vi "Laser.vi"() -> ()   [LabVIEW 2013]
doc: "Пограмма управления мишенью лазерного источника ионов."
uses:
  <vilib>/Utility/error.llb/DialogType.ctl
  <vilib>/Utility/inputDevices.llb/closeMouse.vi
  <vilib>/Utility/inputDevices.llb/mouseAcquire.vi
panel:
  in  "выстрел  Y Графит":u16 step=1
  in  "выстрел X Графит":u16 step=1
  in  "выстрел Y LiF 2":u16 step=1
  in  "выстрел X LiF 2":u16 step=1
  in  "выстрел Y LiF 1":u16 step=1
  in  "выстрел X LiF 1":u16 step=1
  in  "выстрел Y дейт":u16 step=1
  in  "выстрел X дейт":u16 step=1
  in  "xxx":enum32{" Мишени", " Настройки TCP"}(tab)
  in  "Готово!":bool
  in  "Выстрелов до перемотки":u16=5
  out "id мишени":u16
  in  "Выбор - дейтерий":bool
  in  "Счетчик выстрелов:":dbl
  in  "Шаг перехода по Y графит":dbl format="%.1g"
  in  "Шаг перехода по Х графит":dbl format="%.1g"
  in  "Выстрелов в точку  графит":u16=3
  in  "Шаг перехода по Y LiF 2":dbl format="%.1g"
  in  "Шаг перехода по Х LiF 2":dbl format="%.1g"
  in  "Выстрелов в точку  LiF 2":u16=3
  in  "Шаг перехода по Y LiF 1":dbl format="%.1g"
  in  "Шаг перехода по Х LiF 1":dbl format="%.1g"
  in  "Выстрелов в точку LiF 1":u16=3
  in  "Шаг перехода по Y дейт":dbl format="%.1g"
  in  "Шаг перехода по Х дейт":dbl format="%.1g"
  in  "Выстрелов в точку дейтерий":u16=3
  in  "TCP read data":string
  in  "LiF 2":picture
  in  "LiF 1":picture
  in  "Графит":picture
  in  "Дейтерий":picture
  out "Slide X axis":u8(slide) max=100 scale=0.0..100.0
  out "Slide Y axis":u8(slide) max=50 step=1
  in  "Снимок":bool
  out "con err":bool caption="Connect"
  out "Con":bool
  out "warning1":string
  out "Mouse on Pane pos Horizontal":i32
  out "Mouse on Pane pos Vertical":i32
  in  "Выбор - LiF 1":bool
  in  "Выбор - LiF 2":bool
  in  "Выбор -  Графит":bool
  in  "Выстрел по мишени!":u32
  in  "порт":u16=10001
  in  "IP-адрес":string="159.93.126.157"
  in  "Disconnect":bool caption="Disconn"
  out "Connected":bool
  in  "Connect":bool
  out "TCP error source":string
  in  "stop":bool
  out "read_error_indicator":bool
  in  "Connect 2":bool caption="Connect"
  in  "flag1":bool caption="Disconn"
  out "x+1":dbl
  out "TCP con ID":refnum<k5>
  # "LiF 1"
  # "Дейтерированный полиэтилен"
  # "LiF 2"
  # "Графит"
  # "Шаг перехода по Y, мм"
  # "Шаг перехода по Х, мм"
  # "Выстрелов в точку"
  # "Выстрелов в точку"
  # "Шаг перехода по Х, мм"
  # "Шаг перехода по Y, мм"
  # "Выстрелов в точку"
  # "Шаг перехода по Х, мм"
  # "Шаг перехода по Y, мм"
  # "Выстрелов в точку"
  # "Шаг перехода по Х, мм"
  # "Шаг перехода по Y, мм"
  # "LiF 2"
  # "LiF 1"
  # "Графит"
  # "Дейтерированный полиэтилен"
types:
  T1 = typedef "DialogType.ctl" = u16
  T2 = typedef "imagedata.ctl" = cluster{"image type":i32, "image depth":i32, "image":u8[], "mask":u8[], "colors":u32[], "Rectangle":cluster{"left":i16, "top":i16, "right":i16, "bottom":i16}}
  T3 = typedef "LVRectTypeDef.ctl" = cluster{"Left":i16, "Top":i16, "Right":i16, "Bottom":i16}
  T4 = cluster{"Horizontal":i32, "Vertical":i32, "Scrolling":i32}
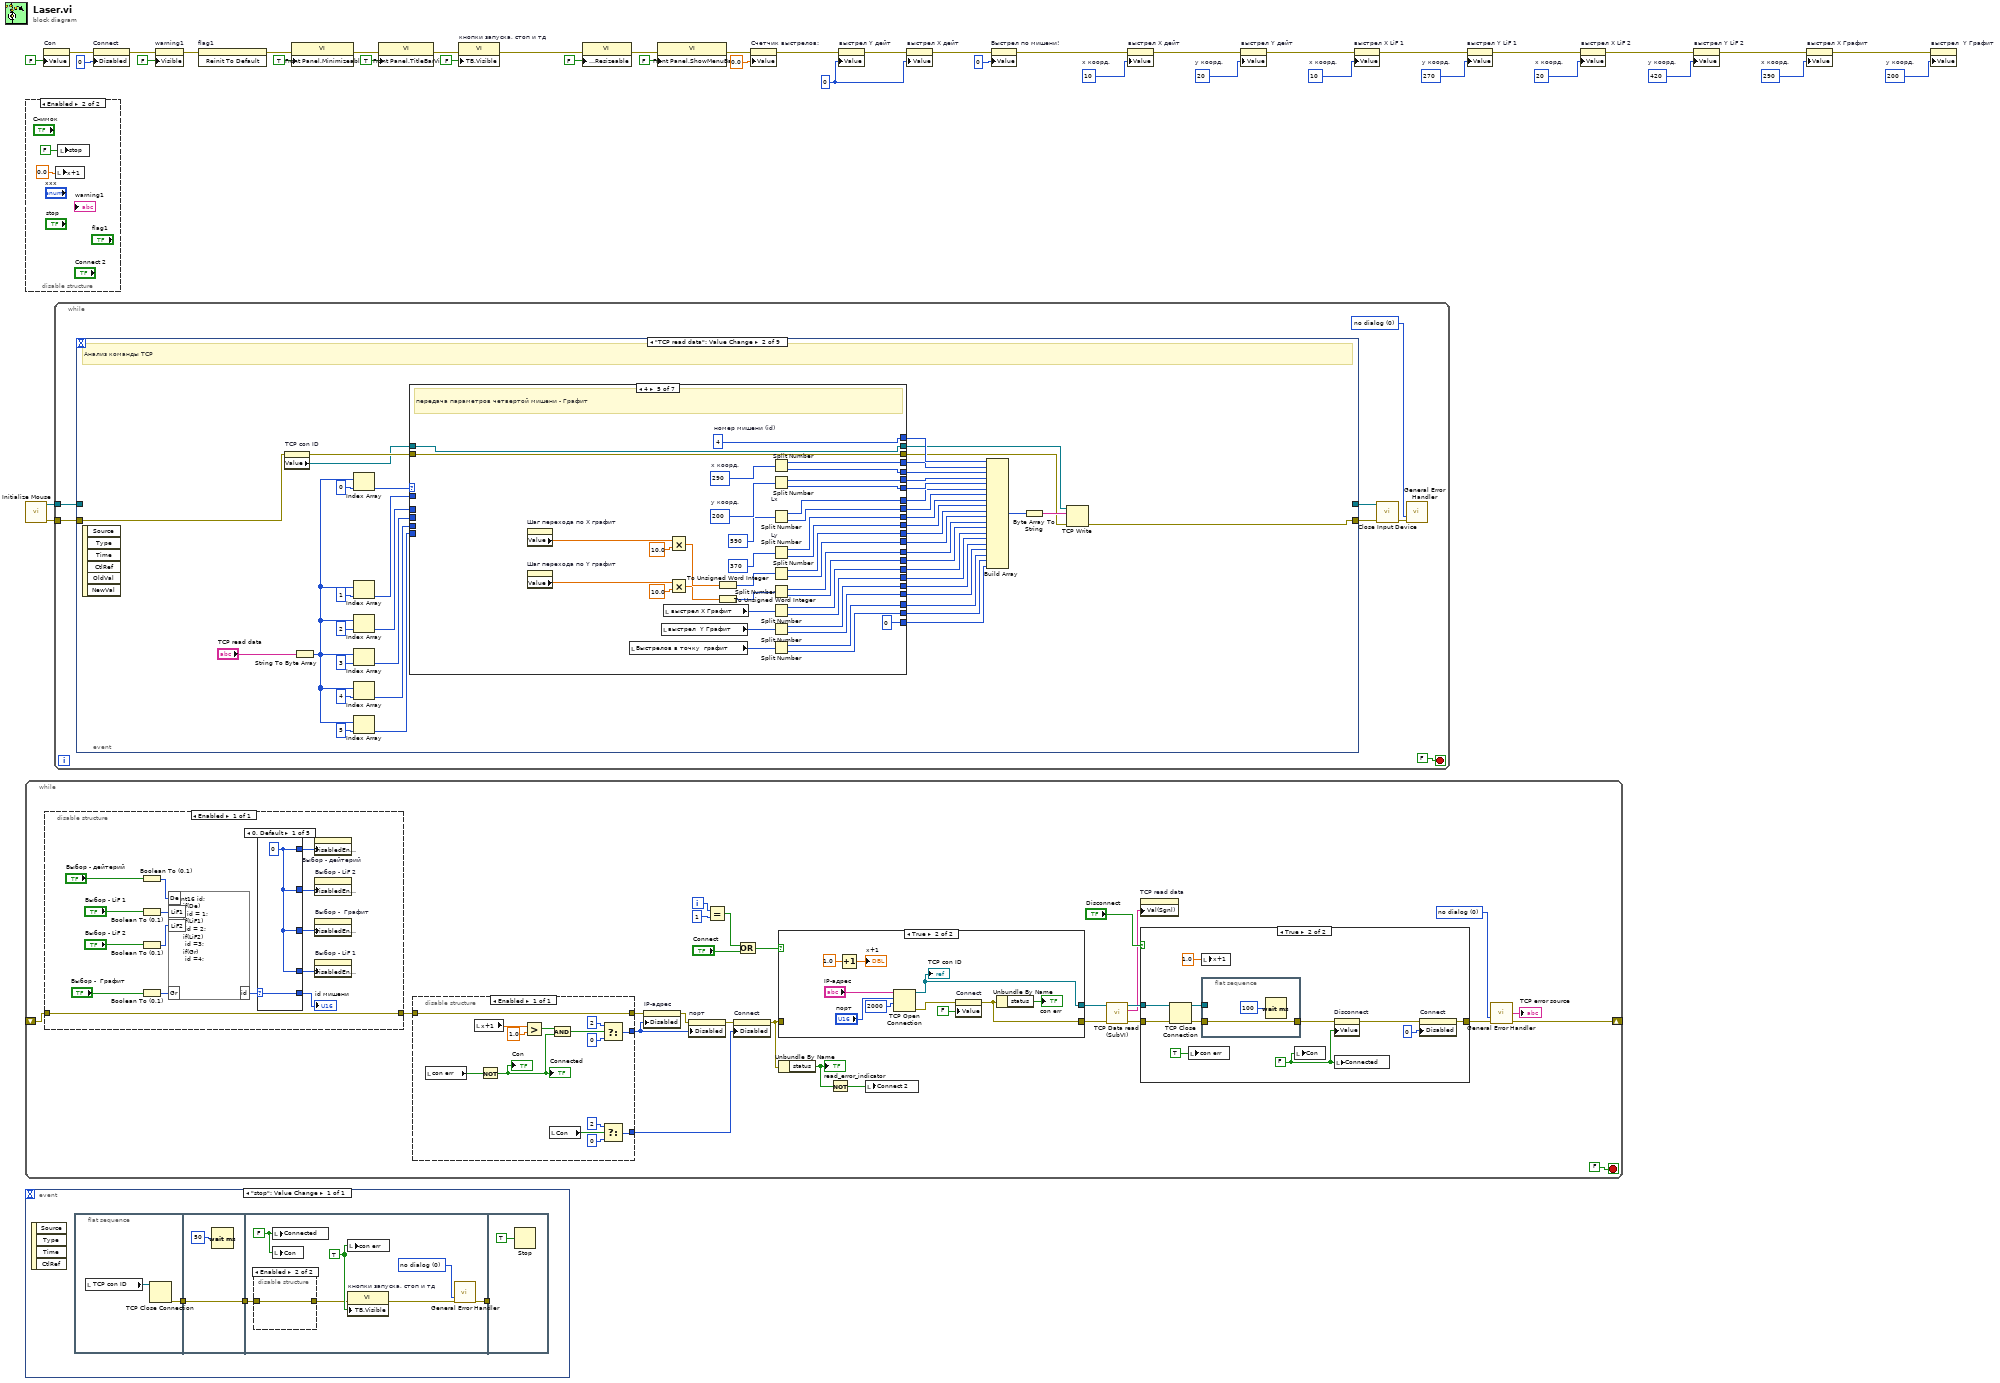
[diagram p0: block diagram]
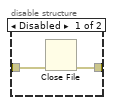
[diagram p3: hidden frame]
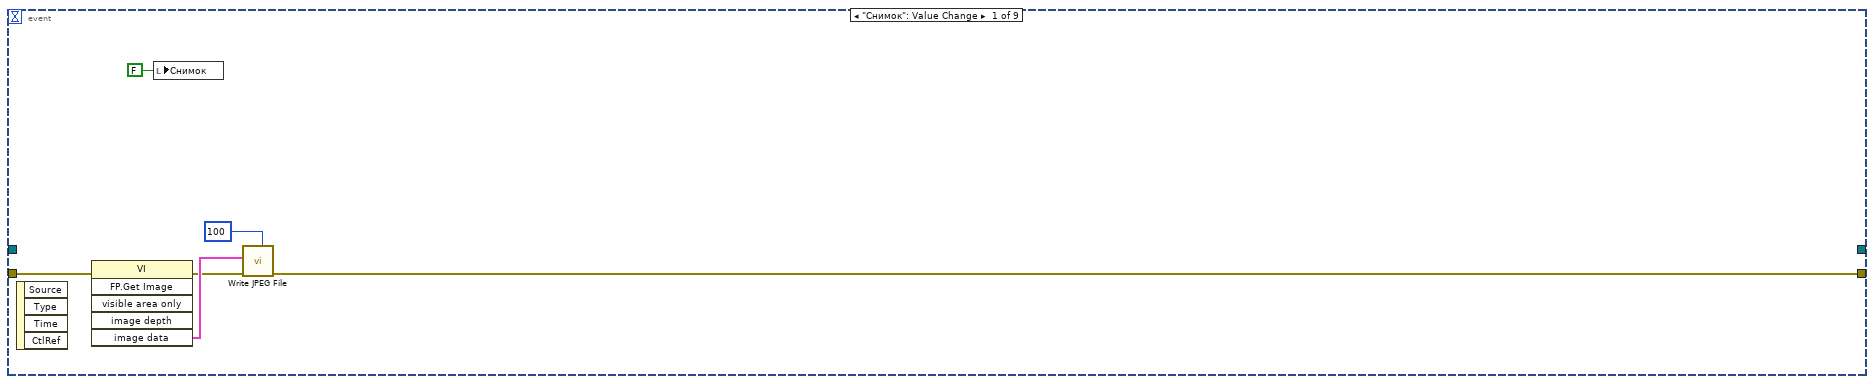
[diagram p4: hidden frame]
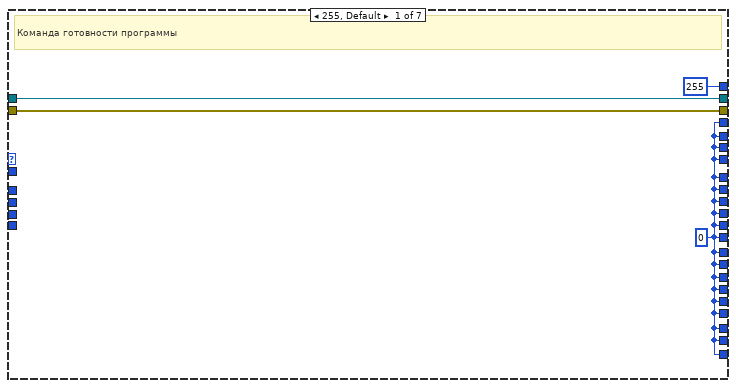
[diagram p5: hidden frame]
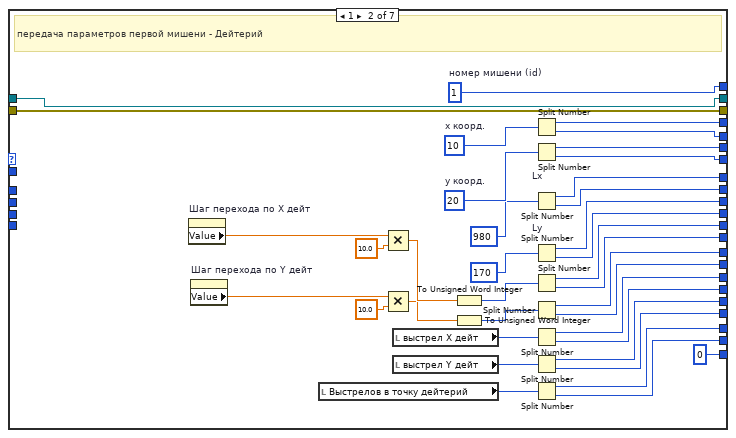
[diagram p6: hidden frame]
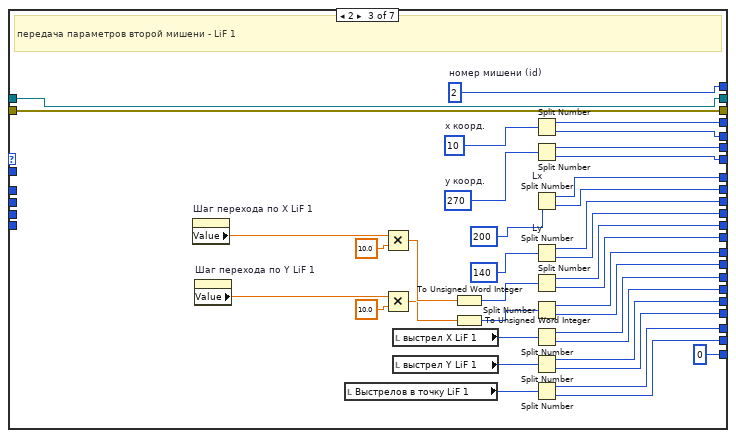
[diagram p7: hidden frame]
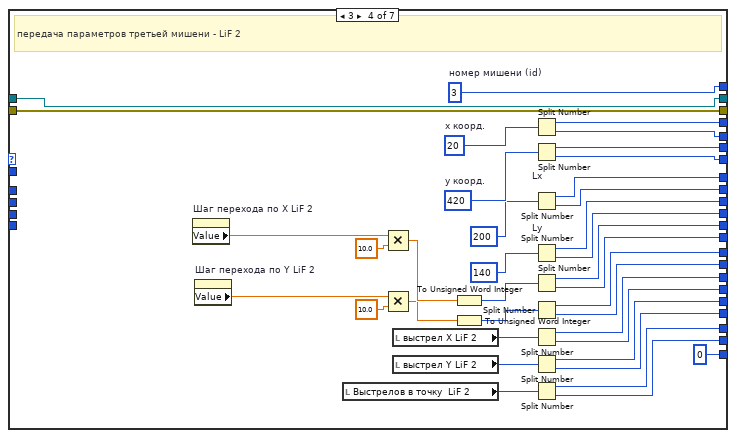
[diagram p8: hidden frame]
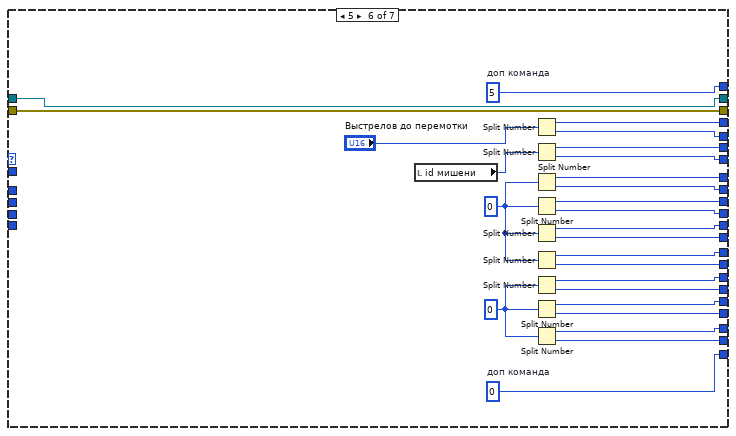
[diagram p9: hidden frame]
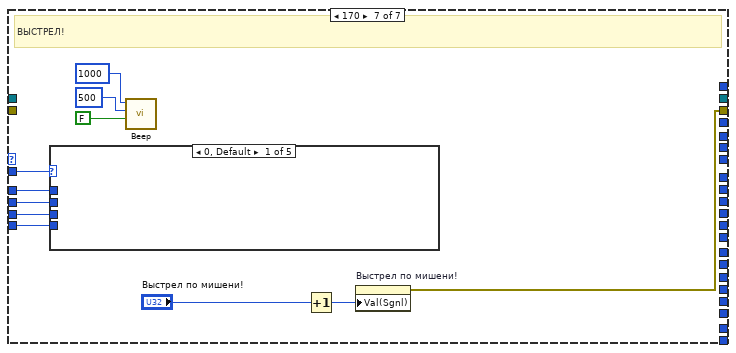
[diagram p10: hidden frame]
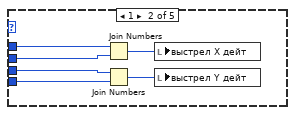
[diagram p11: hidden frame]
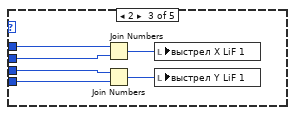
[diagram p12: hidden frame]
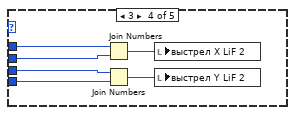
[diagram p13: hidden frame]
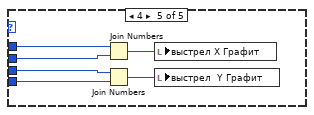
[diagram p14: hidden frame]
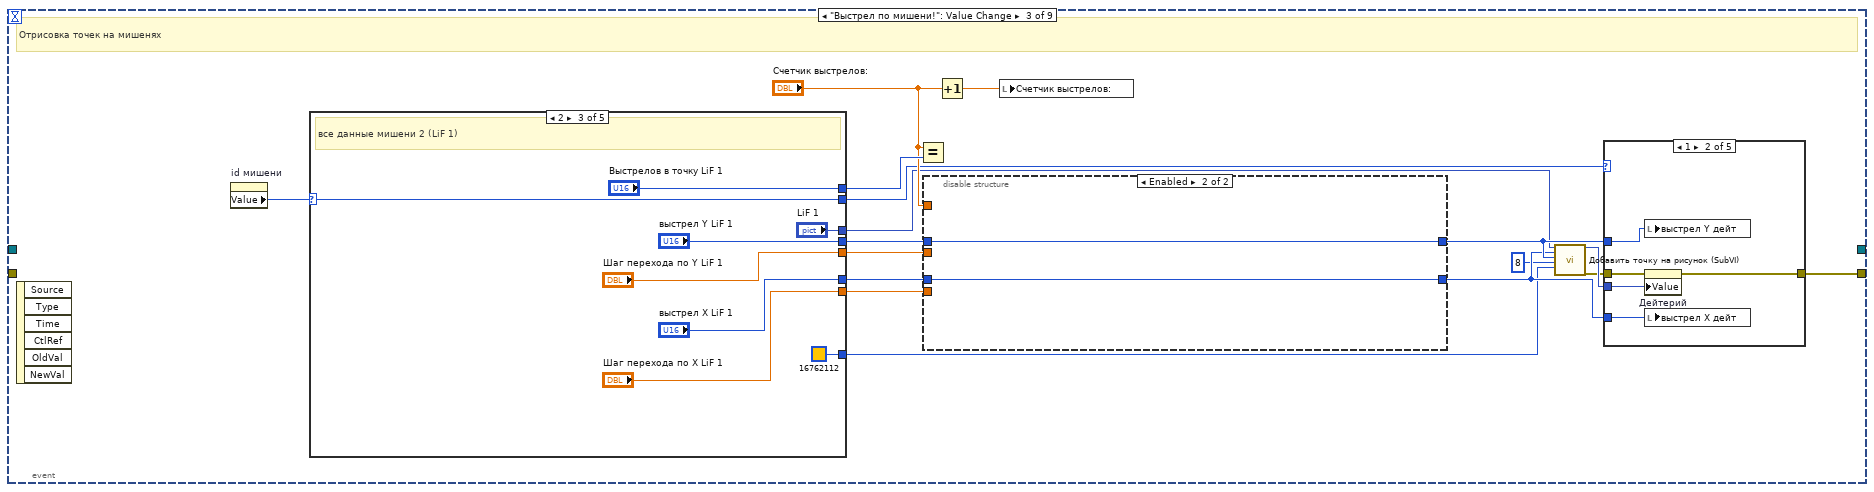
[diagram p15: hidden frame]
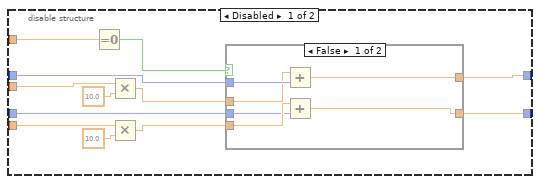
[diagram p16: hidden frame]
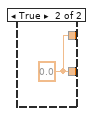
[diagram p17: hidden frame]
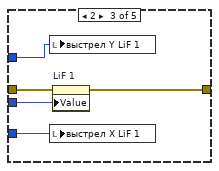
[diagram p19: hidden frame]
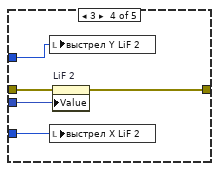
[diagram p20: hidden frame]
diagram:
  w2 = u16 200  # y коорд.
  w3 = u16 290  # x коорд.
  w4 = u16 420  # y коорд.
  w5 = u16 20  # x коорд.
  w6 = u16 270  # y коорд.
  w7 = u16 10  # x коорд.
  w15 = u16 20  # y коорд.
  w16 = u16 10  # x коорд.
  w20 = u16 0 ("выстрел Y дейт")
  n1 = disable-structure shown="Enabled" {
    frame Disabled {
    }
    frame Enabled {
      n2 = local write "x+1"(0.0 ("x+1")) -> ()
      n3 = local write "stop"(FALSE ("Boolean")) -> ()
    }
  }
  n4 = call <vilib>:"Initialize Mouse.vi"() -> ("error out"=w25:errorcluster, "device ID"=w24:refnum<k1>)  [unwired: 1 in, 9 out]
  n5 = while {
    shift-right: [w56] -> _
    shift-left: _ -> [w44]
    i -> [w61]
    stop <- FALSE stop-if-true
    w57 = T1 0 items=["no dialog", "OK message", "continue or stop message", "OK message + warnings", "continue/stop + warnings"] ("type of dialog (OK msg:1)")
    n6 = disable-structure shown="Enabled" {
      disable-tunnel: [w90] -> w45
      disable-tunnel: w44 -> [w90]
      frame Enabled {
        n7 = Boolean To (0,1)(Boolean="Выбор - дейтерий") -> (0, 1=w97:i16)
        n8 = Boolean To (0,1)(Boolean="Выбор - LiF 1") -> (0, 1=w96:i16)
        n9 = Boolean To (0,1)(Boolean="Выбор - LiF 2") -> (0, 1=w95:i16)
        n10 = Boolean To (0,1)(Boolean="Выбор -  Графит") -> (0, 1=w94:i16)
        n11 = formula code="uInt16 id;\n    if(De)\n      id = 1;\n    if(LiF1)\n     id = 2;\n    if(LiF2)\n     id =3;\n    if(Gr)\n     id =4;"("De"=w97, "LiF1"=w96, "LiF2"=w95, "Gr"=w94) -> ("id"=w89:u16)
        n12 = case shown="0, Default" w89 {
          selector: w89 -> [w99 w101 w106 w111 w116]
          tunnel: [w100 u8 0 ("Disabled") u8 2 ("Disabled") u8 2 ("Disabled") u8 2 ("Disabled")] -> w88
          tunnel: [w100 u8 2 ("Disabled") u8 0 ("Disabled") u8 2 ("Disabled") u8 2 ("Disabled")] -> w87
          tunnel: [w100 u8 2 ("Disabled") u8 2 ("Disabled") u8 0 ("Disabled") u8 2 ("Disabled")] -> w86
          tunnel: [w100 u8 2 ("Disabled") u8 2 ("Disabled") u8 2 ("Disabled") u8 0 ("Disabled")] -> w85
          tunnel: [w99 w101 w106 w111 w116] -> w84
          frame 0, Default {
            w100 = u8 0 ("Disabled")
          }
          frame 1 {
          }
          frame 2 {
          }
          frame 3 {
          }
          frame 4 {
          }
        }
        "id мишени" <- w84
        n13 = property on="Выбор - дейтерий" class="Bool (strict)"("DisabledEnum"=w88) -> ()  [unwired: 2 in, 2 out]
        n14 = property on="Выбор - LiF 2" class="Bool (strict)"("DisabledEnum"=w86) -> ()  [unwired: 2 in, 2 out]
        n15 = property on="Выбор -  Графит" class="Bool (strict)"("DisabledEnum"=w85) -> ()  [unwired: 2 in, 2 out]
        n16 = property on="Выбор - LiF 1" class="Bool (strict)"("DisabledEnum"=w87) -> ()  [unwired: 2 in, 2 out]
      }
    }
    n17 = disable-structure shown="Enabled" {
      disable-tunnel: [w75] -> w67
      disable-tunnel: [w71] -> w47
      disable-tunnel: [w70] -> w46
      disable-tunnel: w45 -> [w70]
      frame Enabled {
        n18 = local read "con err"() -> (w80:bool)
        n19 = local read "x+1"() -> (w83:dbl)
        n20 = Not(x=w80) -> (.not. x?=w79:bool)
        "Connected" <- w79
        "Con" <- w79
        n21 = Greater?(x=w83, y=1.0) -> (0:w81:bool)
        n22 = local read "Con"() -> (w72:bool)
        n23 = And(x=w81, y=w79) -> (x .and. y?=w76:bool)
        n24 = Select(t=u8 2 ("Disabled"), s=w76, f=u8 0 ("Disabled")) -> (s? t:f=w75:u8)
        n25 = Select(t=u8 2 ("Disabled"), s=w72, f=u8 0 ("Disabled")) -> (s? t:f=w71:u8)
      }
    }
    n26 = property on="IP-адрес" class="Str"(error in=w46, "Disabled"=w67) -> (error out=w66:errorcluster)  [unwired: 1 in, 1 out]
    n27 = property on="порт" class="DigNum (strict)"(error in=w66, "Disabled"=w67) -> (error out=w65:errorcluster)  [unwired: 1 in, 1 out]
    n28 = Equal?(x=w61, y=1) -> (x = y?=w62:bool)
    n29 = property on="Connect" class="Bool (strict)"(error in=w65, "Disabled"=w47) -> (error out=w59:errorcluster)  [unwired: 1 in, 1 out]
    n30 = Or(x=w62, y="Connect") -> (x .or. y?=w64:bool)
    n31 = case shown="True" w64 {
      tunnel: [w122 w123] -> w53
      tunnel: [w121 w124] -> w51
      tunnel: w59 -> [w122 _]
      frame False {
        n32 = local read "TCP con ID"() -> (w121:refnum<k5>)
      }
      frame True {
        n33 = Increment(x=1.0) -> (x+1=→"x+1":dbl)
        n34 = TCP Open Connection(address="IP-адрес", remote port or service name="порт", timeout ms (60000)=2000) -> (connection ID=w124:refnum<k5>, error out=w126:errorcluster)  [unwired: 1 in, 1 out]
        "TCP con ID" <- w124
        n35 = property on="Connect" class="Bool (strict)"(error in=w126, "Value"=FALSE ("Connect")) -> (error out=w123:errorcluster)  [unwired: 1 in, 1 out]
        n36 = Unbundle By Name(w123) -> ("status"=→"con err":bool)
      }
    }
    n37 = Unbundle By Name(w59) -> ("status"=w54:bool)
    "read_error_indicator" <- w54
    n38 = Not(x=w54) -> (.not. x?=w69:bool)
    n39 = local write "Connect 2"(w69) -> ()
    n40 = call "TCP Data read (SubVI).vi"("error in (no error)"=w53, "TCP Network Connection in"=w51) -> ("error out"=w52:errorcluster, "Read data"=w48:string, "TCP Network Connection out"=w50:refnum<k5>)  [unwired: 1 in, 6 out]
    n41 = property on="TCP read data" class="Str"("Val(Sgnl)"=w48) -> ()  [unwired: 2 in, 2 out]
    n42 = case shown="True" "Disconnect" {
      tunnel: [_ w135] -> w55
      tunnel: w52 -> [_ w134]
      tunnel: w50 -> [_ w133]
      frame False {
      }
      frame True {
        w136 = FALSE ("Disconnect")
        n43 = TCP Close Connection(connection ID=w133, error in (no error)=w134) -> (connection ID out=w139:refnum<k5>, error out=w138:errorcluster)  [unwired: 1 out]
        n44 = local write "con err"(TRUE ("con err")) -> ()
        n45 = local write "x+1"(1.0 ("1")) -> ()
        n46 = flat-sequence {
          tunnel: w139 -> [_]
          tunnel: w138 -> [w144]
          tunnel: [w144] -> w137
          frame #0 {
            n47 = Wait (ms)(milliseconds to wait=u32 100) -> ()  [unwired: 1 out]
          }
        }
        n48 = local write "Con"(w136) -> ()
        n49 = property on="Disconnect" class="Bool (strict)"(error in=w137, "Value"=w136) -> (error out=w140:errorcluster)  [unwired: 1 in, 1 out]
        n50 = local write "Connected"(w136) -> ()
        n51 = property on="Connect" class="Bool (strict)"(error in=w140, "Disabled"=u8 0) -> (error out=w135:errorcluster)  [unwired: 1 in, 1 out]
      }
    }
    n52 = call <vilib>:"General Error Handler.vi"("type of dialog (OK msg:1)"=w57, "error in (no error)"=w55) -> ("source out"=→"TCP error source":string, "error out"=w56:errorcluster)  [unwired: 12 out]
  }
  n53 = event shown="[0] \"stop\": Value Change" {
    selector: _ -> [_]
    dyn-events: _ -> [_]
    timeout: _ -> [_]
    event "stop": Value Change {
      n54 = event-data() -> ()  [unwired: 5 out]
      n55 = flat-sequence {
        tunnel: [w149] -> w148
        tunnel: w148 -> [w152]
        tunnel: [w152] -> w147
        tunnel: w147 -> [w156]
        tunnel: [w154] -> w146
        tunnel: w146 -> [_]
        frame #0 {
          n56 = local read "TCP con ID"() -> (w150:refnum<k5>)
          n57 = TCP Close Connection(connection ID=w150) -> (error out=w149:errorcluster)  [unwired: 1 in, 2 out]
        }
        frame #1 {
          n58 = Wait (ms)(milliseconds to wait=u32 50) -> ()  [unwired: 1 out]
        }
        frame #2 {
          w157 = T1 0 items=["no dialog", "OK message", "continue or stop message", "OK message + warnings", "continue/stop + warnings"] ("type of dialog (OK msg:1)")
          w159 = FALSE ("Запись в файл")
          w158 = TRUE ("Tool Bar:Visible")
          n59 = disable-structure shown="Enabled" {
            disable-tunnel: [w161 w162] -> w153
            disable-tunnel: w156 -> [w160 w162]
            frame Disabled {
              n60 = Close File(error in=w160) -> (error out=w161:errorcluster)  [unwired: 1 in, 1 out]
            }
            frame Enabled {
            }
          }
          n61 = local write "Connected"(w159) -> ()
          n62 = local write "Con"(w159) -> ()
          n63 = local write "con err"(w158) -> ()
          n64 = property on="кнопки запуска, стоп и тд" class="VI"(error in=w153, "TB.Visible"=w158) -> (error out=w155:errorcluster)  [unwired: 1 in, 1 out]
          n65 = call <vilib>:"General Error Handler.vi"("type of dialog (OK msg:1)"=w157, "error in (no error)"=w155) -> ("error out"=w154:errorcluster)  [unwired: 13 out]
        }
        frame #3 {
          n66 = Stop(stop? (T)=TRUE) -> ()
        }
      }
    }
  }
  n67 = property on="Con" class="Bool (strict)"("Value"=FALSE ("Connected")) -> (error out=w28:errorcluster)  [unwired: 2 in, 1 out]
  n68 = while {
    tunnel: w25 -> [w168]
    tunnel: w24 -> [w167]
    stop <- FALSE stop-if-true
    w169 = T1 0 items=["no dialog", "OK message", "continue or stop message", "OK message + warnings", "continue/stop + warnings"] ("type of dialog (OK msg:1)")
    n69 = event shown="[1] \"TCP read data\": Value Change" {
      selector: _ -> [_ _ _ _ _ _ _ _ _]
      dyn-events: _ -> [_ _ _ _ _ _ _ _ _]
      timeout: _ -> [_ _ _ _ _ _ _ _ _]
      tunnel: [w172 w189 w445 w524 w538 w551 w564 w586 w612] -> w166
      tunnel: w168 -> [w171 w217 _ w526 w539 w552 w565 w576 w619]
      tunnel: w167 -> [_ _ _ _ _ _ _ _ w620]
      tunnel: [_ _ _ _ _ _ _ _ w618] -> w164
      event "Снимок": Value Change {
        n70 = event-data() -> ()  [unwired: 5 out]
        n71 = invoke class="VI" method="FP.Get Image"(error in=w171) -> (error out=w173:errorcluster, "image data"=w174:T2)  [unwired: 5 in, 4 out]
        n72 = local write "Снимок"(FALSE ("Снимок")) -> ()
        n73 = call <vilib>:"Write JPEG File.vi"("quality (80)"=100, "error in (no error)"=w173, "image data"=w174) -> ("error out"=w172:errorcluster)  [unwired: 1 in, 7 out]
      }
      event "TCP read data": Value Change {
        # "Анализ команды TCP"
        n74 = event-data() -> ()  [unwired: 7 out]
        n75 = property on="TCP con ID" class="Ref (strict)"(error in=w217) -> (error out=w216:errorcluster, "Value"=w215:refnum<k5>)  [unwired: 1 in, 1 out]
        n76 = String To Byte Array(string="TCP read data") -> (unsigned byte array=w180:u8[])
        n77 = Index Array(array=w180, index=0) -> (element=w214:u8)
        n78 = Index Array(array=w180, index=1) -> (element=w187:u8)
        n79 = Index Array(array=w180, index=2) -> (element=w185:u8)
        n80 = Index Array(array=w180, index=3) -> (element=w183:u8)
        n81 = Index Array(array=w180, index=4) -> (element=w179:u8)
        n82 = Index Array(array=w180, index=5) -> (element=w178:u8)
        n83 = case shown="4" w214 {
          tunnel: w216 -> [w220 w223 w260 w307 w344 w371 _]
          tunnel: w215 -> [w221 w224 w261 w308 w345 w383 _]
          tunnel: [u8 255 ("доп команда") w244 w281 w333 w370 w396 _] -> w211
          tunnel: [w219 w243 w280 w331 w368 w395 _] -> w210
          tunnel: [w219 w242 w279 w330 w367 w394 _] -> w209
          tunnel: [w219 w241 w278 w318 w355 w393 _] -> w208
          tunnel: [w219 w240 w277 w317 w354 w392 _] -> w207
          tunnel: [w219 w239 w276 w316 w353 w391 _] -> w206
          tunnel: [w219 w238 w275 w315 w352 w390 _] -> w205
          tunnel: [w219 w237 w274 w314 w351 w389 _] -> w204
          tunnel: [w219 w236 w273 w313 w350 w388 _] -> w203
          tunnel: [w219 w235 w272 w312 w349 w387 _] -> w202
          tunnel: [w219 w234 w271 w311 w348 w386 _] -> w201
          tunnel: [w219 w232 w270 w310 w347 w385 _] -> w200
          tunnel: [w219 w231 w269 w309 w346 w384 _] -> w199
          tunnel: [w219 u8 0 u8 0 u8 0 ("номер мишени (id)") u8 0 ("номер мишени (id)") w378 _] -> w198
          tunnel: [w219 w230 w267 w305 w342 w382 _] -> w197
          tunnel: [w219 w229 w266 w304 w341 w381 _] -> w196
          tunnel: [w219 w228 w265 w302 w339 w380 _] -> w195
          tunnel: [w219 w227 w264 w301 w338 w379 _] -> w194
          tunnel: [w219 w226 w263 w298 w335 w377 _] -> w193
          tunnel: [w219 w225 w262 w297 w334 w376 _] -> w192
          tunnel: [w221 w224 w261 w308 w345 w383 _] -> w191
          tunnel: [w220 w223 w260 w307 w344 w371 w397] -> w190
          tunnel: w187 -> [_ _ _ _ _ _ w403]
          tunnel: w185 -> [_ _ _ _ _ _ w407]
          tunnel: w183 -> [_ _ _ _ _ _ w406]
          tunnel: w179 -> [_ _ _ _ _ _ w405]
          tunnel: w178 -> [_ _ _ _ _ _ w404]
          frame 255, Default {
            w219 = u8 0
            # "Команда готовности программы"
          }
          frame 1 {
            w244 = u8 1  # номер мишени (id)
            w252 = u16 20  # y коорд.
            w253 = u16 10  # x коорд.
            # "передача параметров первой мишени - Дейтерий"
            n84 = property on="Шаг перехода по Х дейт" class="DigNum (strict)"() -> ("Value"=w259:dbl)  [unwired: 2 in, 2 out]
            n85 = property on="Шаг перехода по Y дейт" class="DigNum (strict)"() -> ("Value"=w256:dbl)  [unwired: 2 in, 2 out]
            n86 = local read "Выстрелов в точку дейтерий"() -> (w245:u16)
            n87 = Multiply(x=w259, y=10.0) -> (x*y=w255:dbl)
            n88 = Multiply(x=w256, y=10.0) -> (x*y=w254:dbl)
            n89 = local read "выстрел X дейт"() -> (w247:u16)
            n90 = local read "выстрел Y дейт"() -> (w246:u16)
            n91 = To Unsigned Word Integer(number=w255) -> (unsigned 16bit integer=w249:u16)
            n92 = To Unsigned Word Integer(number=w254) -> (unsigned 16bit integer=w248:u16)
            n93 = Split Number(x=w253) -> (hi(x)=w243:u8, lo(x)=w242:u8)
            n94 = Split Number(x=w252) -> (hi(x)=w241:u8, lo(x)=w240:u8)
            n95 = Split Number "Lx"(x=u16 980) -> (hi(x)=w239:u8, lo(x)=w238:u8)
            n96 = Split Number "Ly"(x=u16 170) -> (hi(x)=w237:u8, lo(x)=w236:u8)
            n97 = Split Number(x=w249) -> (hi(x)=w235:u8, lo(x)=w234:u8)
            n98 = Split Number(x=w248) -> (hi(x)=w232:u8, lo(x)=w231:u8)
            n99 = Split Number(x=w247) -> (hi(x)=w230:u8, lo(x)=w229:u8)
            n100 = Split Number(x=w246) -> (hi(x)=w228:u8, lo(x)=w227:u8)
            n101 = Split Number(x=w245) -> (hi(x)=w226:u8, lo(x)=w225:u8)
          }
          frame 2 {
            w281 = u8 2  # номер мишени (id)
            w295 = u16 270  # y коорд.
            w296 = u16 10  # x коорд.
            # "передача параметров второй мишени - LiF 1"
            n102 = property on="Шаг перехода по Х LiF 1" class="DigNum (strict)"() -> ("Value"=w288:dbl)  [unwired: 2 in, 2 out]
            n103 = property on="Шаг перехода по Y LiF 1" class="DigNum (strict)"() -> ("Value"=w287:dbl)  [unwired: 2 in, 2 out]
            n104 = local read "Выстрелов в точку LiF 1"() -> (w282:u16)
            n105 = Multiply(x=w288, y=10.0) -> (x*y=w290:dbl)
            n106 = Multiply(x=w287, y=10.0) -> (x*y=w289:dbl)
            n107 = local read "выстрел X LiF 1"() -> (w284:u16)
            n108 = local read "выстрел Y LiF 1"() -> (w283:u16)
            n109 = To Unsigned Word Integer(number=w290) -> (unsigned 16bit integer=w286:u16)
            n110 = To Unsigned Word Integer(number=w289) -> (unsigned 16bit integer=w285:u16)
            n111 = Split Number(x=w296) -> (hi(x)=w280:u8, lo(x)=w279:u8)
            n112 = Split Number(x=w295) -> (hi(x)=w278:u8, lo(x)=w277:u8)
            n113 = Split Number "Lx"(x=u16 200) -> (hi(x)=w276:u8, lo(x)=w275:u8)
            n114 = Split Number "Ly"(x=u16 140) -> (hi(x)=w274:u8, lo(x)=w273:u8)
            n115 = Split Number(x=w286) -> (hi(x)=w272:u8, lo(x)=w271:u8)
            n116 = Split Number(x=w285) -> (hi(x)=w270:u8, lo(x)=w269:u8)
            n117 = Split Number(x=w284) -> (hi(x)=w267:u8, lo(x)=w266:u8)
            n118 = Split Number(x=w283) -> (hi(x)=w265:u8, lo(x)=w264:u8)
            n119 = Split Number(x=w282) -> (hi(x)=w263:u8, lo(x)=w262:u8)
          }
          frame 3 {
            w323 = u16 420  # y коорд.
            w332 = u16 20  # x коорд.
            w333 = u8 3  # номер мишени (id)
            # "передача параметров третьей мишени - LiF 2"
            n120 = property on="Шаг перехода по Х LiF 2" class="DigNum (strict)"() -> ("Value"=w328:dbl)  [unwired: 2 in, 2 out]
            n121 = property on="Шаг перехода по Y LiF 2" class="DigNum (strict)"() -> ("Value"=w329:dbl)  [unwired: 2 in, 2 out]
            n122 = local read "Выстрелов в точку  LiF 2"() -> (w299:u16)
            n123 = Multiply(x=w328, y=10.0) -> (x*y=w325:dbl)
            n124 = Multiply(x=w329, y=10.0) -> (x*y=w324:dbl)
            n125 = local read "выстрел X LiF 2"() -> (w306:u16)
            n126 = local read "выстрел Y LiF 2"() -> (w303:u16)
            n127 = To Unsigned Word Integer(number=w325) -> (unsigned 16bit integer=w320:u16)
            n128 = To Unsigned Word Integer(number=w324) -> (unsigned 16bit integer=w319:u16)
            n129 = Split Number(x=w332) -> (hi(x)=w331:u8, lo(x)=w330:u8)
            n130 = Split Number(x=w323) -> (hi(x)=w318:u8, lo(x)=w317:u8)
            n131 = Split Number "Lx"(x=u16 200) -> (hi(x)=w316:u8, lo(x)=w315:u8)
            n132 = Split Number "Ly"(x=u16 140) -> (hi(x)=w314:u8, lo(x)=w313:u8)
            n133 = Split Number(x=w320) -> (hi(x)=w312:u8, lo(x)=w311:u8)
            n134 = Split Number(x=w319) -> (hi(x)=w310:u8, lo(x)=w309:u8)
            n135 = Split Number(x=w306) -> (hi(x)=w305:u8, lo(x)=w304:u8)
            n136 = Split Number(x=w303) -> (hi(x)=w302:u8, lo(x)=w301:u8)
            n137 = Split Number(x=w299) -> (hi(x)=w298:u8, lo(x)=w297:u8)
          }
          frame 4 {
            w360 = u16 200  # y коорд.
            w369 = u16 290  # x коорд.
            w370 = u8 4  # номер мишени (id)
            # "передача параметров четвертой мишени - Графит"
            n138 = property on="Шаг перехода по Х графит" class="DigNum (strict)"() -> ("Value"=w365:dbl)  [unwired: 2 in, 2 out]
            n139 = property on="Шаг перехода по Y графит" class="DigNum (strict)"() -> ("Value"=w366:dbl)  [unwired: 2 in, 2 out]
            n140 = local read "Выстрелов в точку  графит"() -> (w336:u16)
            n141 = local read "выстрел  Y Графит"() -> (w340:u16)
            n142 = local read "выстрел X Графит"() -> (w343:u16)
            n143 = Multiply(x=w365, y=10.0) -> (x*y=w362:dbl)
            n144 = Multiply(x=w366, y=10.0) -> (x*y=w361:dbl)
            n145 = To Unsigned Word Integer(number=w362) -> (unsigned 16bit integer=w357:u16)
            n146 = To Unsigned Word Integer(number=w361) -> (unsigned 16bit integer=w356:u16)
            n147 = Split Number(x=w369) -> (hi(x)=w368:u8, lo(x)=w367:u8)
            n148 = Split Number(x=w360) -> (hi(x)=w355:u8, lo(x)=w354:u8)
            n149 = Split Number "Lx"(x=u16 590) -> (hi(x)=w353:u8, lo(x)=w352:u8)
            n150 = Split Number "Ly"(x=u16 370) -> (hi(x)=w351:u8, lo(x)=w350:u8)
            n151 = Split Number(x=w357) -> (hi(x)=w349:u8, lo(x)=w348:u8)
            n152 = Split Number(x=w356) -> (hi(x)=w347:u8, lo(x)=w346:u8)
            n153 = Split Number(x=w343) -> (hi(x)=w342:u8, lo(x)=w341:u8)
            n154 = Split Number(x=w340) -> (hi(x)=w339:u8, lo(x)=w338:u8)
            n155 = Split Number(x=w336) -> (hi(x)=w335:u8, lo(x)=w334:u8)
          }
          frame 5 {
            w374 = u16 0
            w378 = u8 0  # доп команда
            w373 = u16 0
            w396 = u8 5  # доп команда
            n156 = local read "id мишени"() -> (w372:u16)
            n157 = Split Number(x="Выстрелов до перемотки") -> (hi(x)=w395:u8, lo(x)=w394:u8)
            n158 = Split Number(x=w372) -> (hi(x)=w393:u8, lo(x)=w392:u8)
            n159 = Split Number ("Lx")(x=w373) -> (hi(x)=w391:u8, lo(x)=w390:u8)
            n160 = Split Number ("Ly")(x=w373) -> (hi(x)=w389:u8, lo(x)=w388:u8)
            n161 = Split Number(x=w373) -> (hi(x)=w387:u8, lo(x)=w386:u8)
            n162 = Split Number(x=w373) -> (hi(x)=w385:u8, lo(x)=w384:u8)
            n163 = Split Number(x=w374) -> (hi(x)=w382:u8, lo(x)=w381:u8)
            n164 = Split Number(x=w374) -> (hi(x)=w380:u8, lo(x)=w379:u8)
            n165 = Split Number(x=w374) -> (hi(x)=w377:u8, lo(x)=w376:u8)
          }
          frame 170 {
            # "ВЫСТРЕЛ!"
            n166 = case shown="0, Default" w403 {
              tunnel: w407 -> [_ w413 w419 w425 w431]
              tunnel: w406 -> [_ w412 w418 w424 w430]
              tunnel: w405 -> [_ w410 w416 w422 w428]
              tunnel: w404 -> [_ w409 w415 w421 w427]
              frame 0, Default {
              }
              frame 1 {
                n167 = Join Numbers(hi=w413, lo=w412) -> ((hi.lo)=w411:u16)
                n168 = Join Numbers(hi=w410, lo=w409) -> ((hi.lo)=w408:u16)
                n169 = local write "выстрел X дейт"(w411) -> ()
                n170 = local write "выстрел Y дейт"(w408) -> ()
              }
              frame 2 {
                n171 = Join Numbers(hi=w419, lo=w418) -> ((hi.lo)=w417:u16)
                n172 = Join Numbers(hi=w416, lo=w415) -> ((hi.lo)=w414:u16)
                n173 = local write "выстрел X LiF 1"(w417) -> ()
                n174 = local write "выстрел Y LiF 1"(w414) -> ()
              }
              frame 3 {
                n175 = Join Numbers(hi=w425, lo=w424) -> ((hi.lo)=w423:u16)
                n176 = Join Numbers(hi=w422, lo=w421) -> ((hi.lo)=w420:u16)
                n177 = local write "выстрел X LiF 2"(w423) -> ()
                n178 = local write "выстрел Y LiF 2"(w420) -> ()
              }
              frame 4 {
                n179 = Join Numbers(hi=w431, lo=w430) -> ((hi.lo)=w429:u16)
                n180 = Join Numbers(hi=w428, lo=w427) -> ((hi.lo)=w426:u16)
                n181 = local write "выстрел X Графит"(w429) -> ()
                n182 = local write "выстрел  Y Графит"(w426) -> ()
              }
            }
            n183 = call <vilib>:"Beep.vi"("use system alert? (T)"=FALSE, "duration (msec)"=u32 500, "frequency (Hz)"=u32 1000) -> ()  [unwired: 9 in]
            n184 = Increment(x="Выстрел по мишени!") -> (x+1=w401:u32)
            n185 = property on="Выстрел по мишени!" class="DigNum (strict)"("Val(Sgnl)"=w401) -> (error out=w397:errorcluster)  [unwired: 2 in, 1 out]
          }
        }
        n186 = Build Array(w211, w210, w209, w208, w207, w206, w205, w204, w203, w202, w201, w200, w199, w197, w196, w195, w194, w193, w192, w198) -> (w213:u8[])
        n187 = Byte Array To String(unsigned byte array=w213) -> (string=w212:string)
        n188 = TCP Write(connection ID=w191, data in=w212, error in (no error)=w190) -> (error out=w189:errorcluster)  [unwired: 1 in, 2 out]
      }
      event "Выстрел по мишени!": Value Change {
        # "Отрисовка точек на мишенях"
        n189 = event-data() -> ()  [unwired: 7 out]
        n190 = property on="id мишени" class="DigNum (strict)"() -> ("Value"=w437:u16)  [unwired: 2 in, 2 out]
        n191 = case shown="2" w437 {
          selector: w437 -> [w491 w492 w500 w515 w522]
          tunnel: [_ "Шаг перехода по Х дейт" "Шаг перехода по Х LiF 1" "Шаг перехода по Х LiF 2" "Шаг перехода по Y графит"] -> w448
          tunnel: [_ "выстрел Y дейт" "выстрел Y LiF 1" "выстрел Y LiF 2" "выстрел  Y Графит"] -> w447
          tunnel: [_ "Шаг перехода по Y дейт" "Шаг перехода по Y LiF 1" "Шаг перехода по Y LiF 2" "Шаг перехода по Х графит"] -> w435
          tunnel: [_ "выстрел X дейт" "выстрел X LiF 1" "выстрел X LiF 2" "выстрел X Графит"] -> w443
          tunnel: [_ "Выстрелов в точку дейтерий" "Выстрелов в точку LiF 1" "Выстрелов в точку  LiF 2" "Выстрелов в точку  графит"] -> w441
          tunnel: [_ "Дейтерий" "LiF 1" "LiF 2" "Графит"] -> w438
          tunnel: [_ u32 3381759 ("цвет") u32 16762112 ("цвет") u32 16762112 ("цвет") u32 9567230 ("цвет")] -> w436
          tunnel: [w491 w492 w500 w515 w522] -> w434
          frame 0, Default {
          }
          frame 1 {
            # "все данный мишени 1 (дейтерий)"
          }
          frame 2 {
            # "все данные мишени 2 (LiF 1)"
          }
          frame 3 {
            # "все данные мишени 3 (LiF 2)"
          }
          frame 4 {
            # "все данные мишени 4 (Графит)"
          }
        }
        n192 = Equal?(x="Счетчик выстрелов:", y=w441) -> ()  [unwired: 1 out]
        n193 = disable-structure shown="Enabled" {
          disable-tunnel: w448 -> [w460 _]
          disable-tunnel: w447 -> [w459 w468]
          disable-tunnel: [w457 w468] -> w446
          disable-tunnel: w443 -> [w454 w469]
          disable-tunnel: [w453 w469] -> w442
          disable-tunnel: "Счетчик выстрелов:" -> [w452 _]
          disable-tunnel: w435 -> [w450 _]
          frame Disabled {
            n194 = Equal To 0?(x=w452) -> (x = 0?=w456:bool)
            n195 = Multiply(x=w450, y=10.0) -> (x*y=w449:dbl)
            n196 = Multiply(x=w460, y=10.0) -> (x*y=w455:dbl)
            n197 = case shown="False" w456 {
              tunnel: w459 -> [w466 _]
              tunnel: w449 -> [w465 _]
              tunnel: [w461 w467] -> w457
              tunnel: w455 -> [w464 _]
              tunnel: w454 -> [w463 _]
              tunnel: [w462 w467] -> w453
              frame False {
                n198 = Add(x=w465, y=w466) -> (x+y=w461:dbl)
                n199 = Add(x=w464, y=w463) -> (x+y=w462:dbl)
              }
              frame True {
                w467 = 0.0
              }
            }
          }
          frame Enabled {
          }
        }
        n200 = Increment(x="Счетчик выстрелов:") -> (x+1=w444:dbl)
        n201 = local write "Счетчик выстрелов:"(w444) -> ()
        n202 = call "Добавить точку на рисунок (SubVI).vi"("in picture"=w438, "dot х"=w442, "dot y"=w446, "thickness"=u16 8, "цвет"=w436) -> ("out picture"=w433:picture, "error out"=w432:errorcluster)  [unwired: 13 in]
        n203 = case shown="1" w434 {
          tunnel: w446 -> [_ w475 w477 w483 w486]
          tunnel: [w470 w471 w476 w481 w489] -> w445
          tunnel: w442 -> [_ w474 w478 w482 w487]
          tunnel: w433 -> [_ w473 w480 w484 w488]
          tunnel: w432 -> [w470 w472 w479 w485 w490]
          frame 0, Default {
          }
          frame 1 {
            n204 = local write "выстрел Y дейт"(w475) -> ()
            n205 = property on="Дейтерий" class="Pict"(error in=w472, "Value"=w473) -> (error out=w471:errorcluster)  [unwired: 1 in, 1 out]
            n206 = local write "выстрел X дейт"(w474) -> ()
          }
          frame 2 {
            n207 = local write "выстрел Y LiF 1"(w477) -> ()
            n208 = local write "выстрел X LiF 1"(w478) -> ()
            n209 = property on="LiF 1" class="Pict"(error in=w479, "Value"=w480) -> (error out=w476:errorcluster)  [unwired: 1 in, 1 out]
          }
          frame 3 {
            n210 = local write "выстрел Y LiF 2"(w483) -> ()
            n211 = local write "выстрел X LiF 2"(w482) -> ()
            n212 = property on="LiF 2" class="Pict"(error in=w485, "Value"=w484) -> (error out=w481:errorcluster)  [unwired: 1 in, 1 out]
          }
          frame 4 {
            n213 = local write "выстрел  Y Графит"(w486) -> ()
            n214 = property on="Графит" class="Pict"(error in=w490, "Value"=w488) -> (error out=w489:errorcluster)  [unwired: 1 in, 1 out]
            n215 = local write "выстрел X Графит"(w487) -> ()
          }
        }
      }
      event "Дейтерий": Shortcut Menu Selection (User) {
        n216 = event-data() -> ("ItemTag"=w525:string)  [unwired: 8 out]
        n217 = case shown="\"Очистить!\"" w525 {
          tunnel: w526 -> [w527 w529]
          tunnel: [w527 w528] -> w524
          frame "False", Default {
            (unwired) FALSE ("Boolean")
          }
          frame "Очистить!" {
            n218 = Two Button Dialog(message="Вы уверены, что хотите очистить эту мишень?", 1:"Нет" ("F button name (\"Cancel\")"), 2:"Да" ("T button name (\"OK\")")) -> (T button?=w530:bool)
            n219 = case shown="True" w530 {
              tunnel: w529 -> [w534 w536]
              tunnel: [w534 w536] -> w528
              frame False {
              }
              frame True {
                n220 = call "Empty Picture"() -> ("empty picture"=w535:picture)
                n221 = local write "Дейтерий"(w535) -> ()
              }
            }
          }
        }
      }
      event "LiF 1": Shortcut Menu Selection (User) {
        # "Очистка мишеней"
        n222 = event-data() -> ("ItemTag"=w537:string)  [unwired: 8 out]
        n223 = case shown="\"Очистить!\"" w537 {
          tunnel: w539 -> [w540 w542]
          tunnel: [w540 w541] -> w538
          frame "False", Default {
          }
          frame "Очистить!" {
            n224 = Two Button Dialog(message="Вы уверены, что хотите очистить эту мишень?", 1:"Нет" ("F button name (\"Cancel\")"), 2:"Да" ("T button name (\"OK\")")) -> (T button?=w543:bool)
            n225 = case shown="True" w543 {
              tunnel: w542 -> [w547 w549]
              tunnel: [w547 w549] -> w541
              frame False {
              }
              frame True {
                n226 = call "Empty Picture"() -> ("empty picture"=w548:picture)
                n227 = local write "LiF 1"(w548) -> ()
              }
            }
          }
        }
      }
      event "LiF 2": Shortcut Menu Selection (User) {
        # "Очистка мишеней"
        n228 = event-data() -> ("ItemTag"=w550:string)  [unwired: 8 out]
        n229 = case shown="\"Очистить!\"" w550 {
          tunnel: w552 -> [w553 w555]
          tunnel: [w553 w554] -> w551
          frame "False", Default {
          }
          frame "Очистить!" {
            n230 = Two Button Dialog(message="Вы уверены, что хотите очистить эту мишень?", 1:"Нет" ("F button name (\"Cancel\")"), 2:"Да" ("T button name (\"OK\")")) -> (T button?=w556:bool)
            n231 = case shown="True" w556 {
              tunnel: w555 -> [w560 w562]
              tunnel: [w560 w562] -> w554
              frame False {
              }
              frame True {
                n232 = call "Empty Picture"() -> ("empty picture"=w561:picture)
                n233 = local write "LiF 2"(w561) -> ()
              }
            }
          }
        }
      }
      event "Графит": Shortcut Menu Selection (User) {
        # "Очистка мишеней"
        n234 = event-data() -> ("ItemTag"=w563:string)  [unwired: 8 out]
        n235 = case shown="\"Очистить!\"" w563 {
          tunnel: w565 -> [w566 w568]
          tunnel: [w566 w567] -> w564
          frame "False", Default {
          }
          frame "Очистить!" {
            n236 = Two Button Dialog(message="Вы уверены, что хотите очистить эту мишень?", 1:"Нет" ("F button name (\"Cancel\")"), 2:"Да" ("T button name (\"OK\")")) -> (T button?=w569:bool)
            n237 = case shown="True" w569 {
              tunnel: w568 -> [w573 w575]
              tunnel: [w573 w575] -> w567
              frame False {
              }
              frame True {
                n238 = call "Empty Picture"() -> ("empty picture"=w574:picture)
                n239 = local write "Графит"(w574) -> ()
              }
            }
          }
        }
      }
      event "Готово!": Value Change {
        w585 = u8 0 ("element")
        # "обновление информации по мишеням"
        n240 = event-data() -> ()  [unwired: 7 out]
        n241 = property on="Готово!" class="Bool (strict)"(error in=w576, "Label.Visible"=TRUE ("Visible")) -> (error out=w578:errorcluster)  [unwired: 1 in, 1 out]
        n242 = flat-sequence {
          tunnel: [w592] -> w579
          tunnel: w578 -> [w592]
          frame #0 {
            n243 = Wait (ms)(milliseconds to wait=u32 300) -> ()  [unwired: 1 out]
          }
        }
        n244 = property on="Готово!" class="Bool (strict)"(error in=w579, "Label.Visible"=FALSE ("Visible")) -> (error out=w577:errorcluster)  [unwired: 1 in, 1 out]
        n245 = property on="Готово!" class="Bool (strict)"(error in=w577, "Value"=FALSE ("обновить данные")) -> (error out=w583:errorcluster)  [unwired: 1 in, 1 out]
        n246 = property on="TCP con ID" class="Ref (strict)"(error in=w583) -> (error out=w588:errorcluster, "Value"=w587:refnum<k5>)  [unwired: 1 in, 1 out]
        n247 = Build Array(u8 85 ("element"), w585, w585, w585, w585, w585, w585, w585, w585, w585, w585, w585, w585, w585, w585, w585, w585, w585, w585, w585) -> (w589:u8[])
        n248 = Byte Array To String(unsigned byte array=w589) -> (string=w584:string)
        n249 = TCP Write(connection ID=w587, data in=w584, error in (no error)=w588) -> (error out=w586:errorcluster)  [unwired: 1 in, 2 out]
      }
      event Mouse Move {
        n250 = event-data() -> ()  [unwired: 6 out]
        n251 = control-ref of="This VI"() -> (w616:refnum<vi>)
        n252 = property class="VI"(reference=w616) -> ("Front Panel.PanelBounds"=w615:T3)  [unwired: 1 in, 2 out]
        n253 = Unbundle By Name(w615) -> ("Left"=w614:i16, "Top"=w613:i16)
        n254 = call-poly <vilib>:"Acquire Input Data.vi"("device ID"=w620, "error in (no error)"=w619) -> ("device ID"=w618:refnum<k1>, "axis info"=w617:T4, "error out"=w612:errorcluster)  [unwired: 1 in, 14 out]
        n255 = Unbundle By Name(w617) -> ("Horizontal"=w610:i32, "Vertical"=w608:i32)
        n256 = To Unsigned Long Integer(number=w614) -> (unsigned 32bit integer=w611:u32)
        n257 = To Unsigned Long Integer(number=w613) -> (unsigned 32bit integer=w609:u32)
        n258 = Subtract(x=w610, y=w611) -> (x-y=w607:u32)
        n259 = Subtract(x=w608, y=w609) -> (x-y=w606:u32)
        n260 = expression code="(x-50)/10" "сдвигаем 0 коорд. по X и приводим к мм"(w607) -> (w601:u32)
        n261 = expression code="(x-47)/10" "сдвигаем 0 коорд. по Y и приводим к мм"(w606) -> (w600:u32)
        n262 = Greater?(x=w600, y=60) -> (0:w598:bool)
        n263 = Greater?(x=w601, y=100) -> (0:w597:bool)
        n264 = Or(x=w597, y=w598) -> (x .or. y?=w599:bool)
        n265 = Select(t=0, s=w599, f=w600) -> (s? t:f=w594:u32)
        "Mouse on Pane pos Vertical" <- w594
        "Slide Y axis" <- w594
        n266 = Equal To 0?(x=w594) -> (x = 0?=w596:bool)
        n267 = Compound Arithmetic op=OR(w598, w597, w596) -> (w595:bool)
        n268 = Select(t=0, s=w595, f=w601) -> (s? t:f=→"Mouse on Pane pos Horizontal" →"Slide X axis":u32)
      }
    }
    n269 = call-poly <vilib>:"Close Input Device.vi"("error in (no error)"=w166, "device ID"=w164) -> ("error out"=w165:errorcluster)  [unwired: 8 out]
    n270 = call <vilib>:"General Error Handler.vi"("type of dialog (OK msg:1)"=w169, "error in (no error)"=w165) -> ()  [unwired: 14 out]
  }
  n271 = property on="Connect" class="Bool (strict)"(error in=w28, "Disabled"=u8 0) -> (error out=w33:errorcluster)  [unwired: 1 in, 1 out]
  n272 = property on="warning1" class="Str"(error in=w33, "Visible"=FALSE) -> (error out=w26:errorcluster)  [unwired: 1 in, 1 out]
  n273 = invoke on="flag1" class="Bool (strict)" method="Reinit To Default"(error in=w26) -> (error out=w27:errorcluster)  [unwired: 2 in, 2 out]
  n274 = property class="VI"(error in=w27, "Front Panel.Minimizeable"=TRUE ("Front Panel Window:Minimizable")) -> (error out=w32:errorcluster)  [unwired: 1 in, 1 out]
  n275 = property class="VI"(error in=w32, "Front Panel.TitleBarVis"=TRUE ("Front Panel Window:Title Bar Visible")) -> (error out=w31:errorcluster)  [unwired: 1 in, 1 out]
  n276 = property on="кнопки запуска, стоп и тд" class="VI"(error in=w31, "TB.Visible"=FALSE ("Tool Bar:Visible")) -> (error out=w30:errorcluster)  [unwired: 1 in, 1 out]
  n277 = property class="VI"(error in=w30, "Front Panel.Resizeable"=FALSE ("Front Panel Window:Resizable")) -> (error out=w29:errorcluster)  [unwired: 1 in, 1 out]
  n278 = property class="VI"(error in=w29, "Front Panel.ShowMenuBar"=FALSE ("Front Panel Window:Show Menu Bar")) -> (error out=w22:errorcluster)  [unwired: 1 in, 1 out]
  n279 = property on="Счетчик выстрелов:" class="DigNum (strict)"(error in=w22, "Value"=0.0 ("Счетчик выстрелов:")) -> (error out=w19:errorcluster)  [unwired: 1 in, 1 out]
  n280 = property on="выстрел Y дейт" class="DigNum (strict)"(error in=w19, "Value"=w20) -> (error out=w21:errorcluster)  [unwired: 1 in, 1 out]
  n281 = property on="выстрел X дейт" class="DigNum (strict)"(error in=w21, "Value"=w20) -> (error out=w1:errorcluster)  [unwired: 1 in, 1 out]
  n282 = property on="Выстрел по мишени!" class="DigNum (strict)"(error in=w1, "Value"=u32 0 ("Выстрел по мишени!")) -> (error out=w14:errorcluster)  [unwired: 1 in, 1 out]
  n283 = property on="выстрел X дейт" class="DigNum (strict)"(error in=w14, "Value"=w16) -> (error out=w17:errorcluster)  [unwired: 1 in, 1 out]
  n284 = property on="выстрел Y дейт" class="DigNum (strict)"(error in=w17, "Value"=w15) -> (error out=w12:errorcluster)  [unwired: 1 in, 1 out]
  n285 = property on="выстрел X LiF 1" class="DigNum (strict)"(error in=w12, "Value"=w7) -> (error out=w13:errorcluster)  [unwired: 1 in, 1 out]
  n286 = property on="выстрел Y LiF 1" class="DigNum (strict)"(error in=w13, "Value"=w6) -> (error out=w10:errorcluster)  [unwired: 1 in, 1 out]
  n287 = property on="выстрел X LiF 2" class="DigNum (strict)"(error in=w10, "Value"=w5) -> (error out=w11:errorcluster)  [unwired: 1 in, 1 out]
  n288 = property on="выстрел Y LiF 2" class="DigNum (strict)"(error in=w11, "Value"=w4) -> (error out=w8:errorcluster)  [unwired: 1 in, 1 out]
  n289 = property on="выстрел X Графит" class="DigNum (strict)"(error in=w8, "Value"=w3) -> (error out=w9:errorcluster)  [unwired: 1 in, 1 out]
  n290 = property on="выстрел  Y Графит" class="DigNum (strict)"(error in=w9, "Value"=w2) -> ()  [unwired: 1 in, 2 out]
